vi "Eulergcd.vi"(8 "b":i32, 11 "a":i32) -> (2 "r":i32)   [LabVIEW 2017]
doc: "this Vi will recieve two positive inteers and return the greatest common divisor"
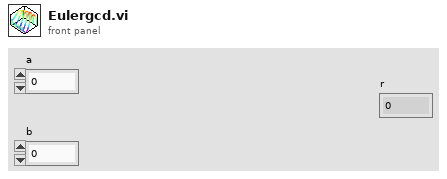
[diagram p1: front panel]
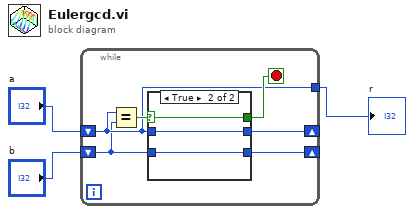
[diagram p0: block diagram]
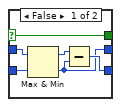
[diagram p2: hidden frame]
diagram:
  n1 = while {
    shift-right: [w5] -> _
    shift-left: "a" -> [w7]
    shift-right: [w4] -> _
    shift-left: "b" -> [w6]
    tunnel: [w7] -> w1
    stop <- w8 stop-if-true
    n2 = Equal?(x=w7, y=w6) -> (x = y?=w9:bool)
    n3 = case shown="True" w9 {
      selector: w9 -> [w12 w18]
      tunnel: [w12 w18] -> w8
      tunnel: w7 -> [w15 w16]
      tunnel: w6 -> [w14 w17]
      tunnel: [w10 w16] -> w5
      tunnel: [w13 w17] -> w4
      frame False {
        n4 = Max & Min(x=w15, y=w14) -> (max(x,y)=w11:i32, min(x,y)=w10:i32)
        n5 = Subtract(x=w11, y=w10) -> (x-y=w13:i32)
      }
      frame True {
      }
    }
  }
  "r" <- w1
